vi "Read vision info keys.vi"() -> ()   [LabVIEW 2020]
panel:
  out "SpatialCalibrationY":T1
  out "error out":errorcluster
  out "Exposure":T1
  out "ROI":T2={"Width"={"Value"=618.0, "Min"=1.0, "Max"=3000.0, "StepSize"=1.0, "Tolerance"=0.0, "valueactual"=0.0}, "Height"={"Value"=813.0, "Min"=1.0, "Max"=3000.0, "StepSize"=1.0, "Tolerance"=0.0, "valueactual"=0.0}, "OffsetX"={"Value"=0.0, "Min"=0.0, "Max"=1000.0, "StepSize"=1.0, "Tolerance"=0.0, "valueactual"=0.0}, "OffsetY"={"Value"=0.0, "Min"=0.0, "Max"=1000.0, "StepSize"=1.0, "Tolerance"=0.0, "valueactual"=0.0}}
  out "SpatialCalibration":T1
  out "Keys":string[](array[string])
  in  "Image path":path
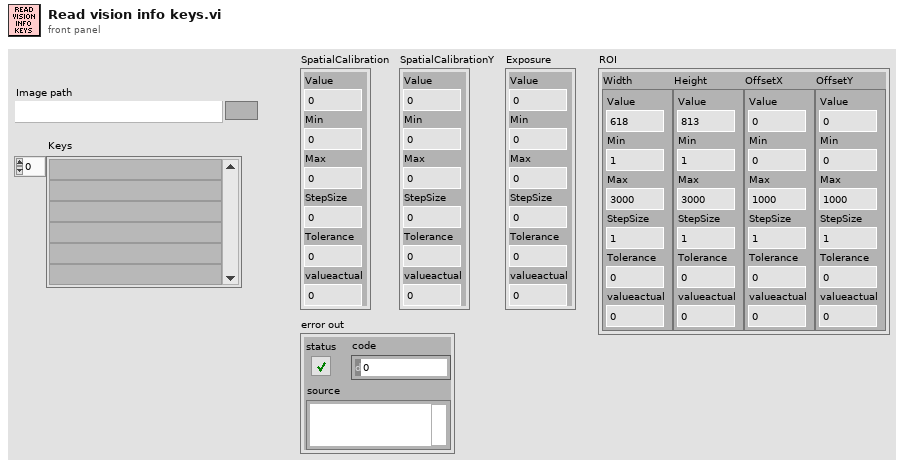
[diagram p1: front panel]
types:
  T1 = cluster{"Value":dbl, "Min":dbl, "Max":dbl, "StepSize":dbl, "Tolerance":dbl, "valueactual":dbl}
  T2 = cluster{"Width":cluster{"Value":dbl, "Min":dbl, "Max":dbl, "StepSize":dbl, "Tolerance":dbl, "valueactual":dbl}, "Height":cluster{"Value":dbl, "Min":dbl, "Max":dbl, "StepSize":dbl, "Tolerance":dbl, "valueactual":dbl}, "OffsetX":cluster{"Value":dbl, "Min":dbl, "Max":dbl, "StepSize":dbl, "Tolerance":dbl, "valueactual":dbl}, "OffsetY":cluster{"Value":dbl, "Min":dbl, "Max":dbl, "StepSize":dbl, "Tolerance":dbl, "valueactual":dbl}}
  T3 = cluster{"SpatialCalibration":cluster{"Value":dbl, "Min":dbl, "Max":dbl, "StepSize":dbl, "Tolerance":dbl, "valueactual":dbl}, "SpatialCalibrationY":cluster{"Value":dbl, "Min":dbl, "Max":dbl, "StepSize":dbl, "Tolerance":dbl, "valueactual":dbl}, "ROI":cluster{"Width":cluster{"Value":dbl, "Min":dbl, "Max":dbl, "StepSize":dbl, "Tolerance":dbl, "valueactual":dbl}, "Height":cluster{"Value":dbl, "Min":dbl, "Max":dbl, "StepSize":dbl, "Tolerance":dbl, "valueactual":dbl}, "OffsetX":cluster{"Value":dbl, "Min":dbl, "Max":dbl, "StepSize":dbl, "Tolerance":dbl, "valueactual":dbl}, "OffsetY":cluster{"Value":dbl, "Min":dbl, "Max":dbl, "StepSize":dbl, "Tolerance":dbl, "valueactual":dbl}}, "Exposure":cluster{"Value":dbl, "Min":dbl, "Max":dbl, "StepSize":dbl, "Tolerance":dbl, "valueactual":dbl}}
  T4 = typedef "IMAQ Image.ctl" = refnum<image>
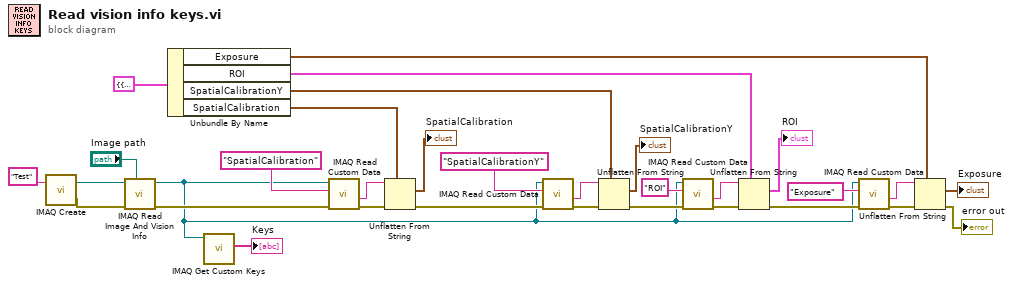
[diagram p0: block diagram]
diagram:
  n1 = call "IMAQ Create"("Image Name"="Test") -> ("New Image"=w30:T4, "error out"=w31:errorcluster)  [unwired: 4 in]
  n2 = call "IMAQ Read Image And Vision Info"("File Path"="Image path", "error in (no error)"=w31, "Image"=w30) -> ("error out"=w23:errorcluster, "Image Out"=w1:T4)  [unwired: 6 in, 1 out]
  n3 = Unbundle By Name(T3 {"SpatialCalibration"={"Value"=0.0, "Min"=0.0, "Max"=0.0, "StepSize"=0.0, "Tolerance"=0.0, "valueactual"=0.0}, "SpatialCalibrationY"={"Value"=0.0, "Min"=0.0, "Max"=0.0, "StepSize"=0.0, "Tolerance"=0.0, "valueactual"=0.0}, "ROI"={"Width"={"Value"=618.0, "Min"=1.0, "Max"=3000.0, "StepSize"=1.0, "Tolerance"=0.0, "valueactual"=0.0}, "Height"={"Value"=813.0, "Min"=1.0, "Max"=3000.0, "StepSize"=1.0, "Tolerance"=0.0, "valueactual"=0.0}, "OffsetX"={"Value"=0.0, "Min"=0.0, "Max"=1000.0, "StepSize"=1.0, "Tolerance"=0.0, "valueactual"=0.0}, "OffsetY"={"Value"=0.0, "Min"=0.0, "Max"=1000.0, "StepSize"=1.0, "Tolerance"=0.0, "valueactual"=0.0}}, "Exposure"={"Value"=0.0, "Min"=0.0, "Max"=0.0, "StepSize"=0.0, "Tolerance"=0.0, "valueactual"=0.0}}) -> ("Exposure"=w12:T1, "ROI"=w17:T2, "SpatialCalibrationY"=w4:T1, "SpatialCalibration"=w5:T1)
  n4 = call "IMAQ Get Custom Keys"("Image"=w1) -> ("Keys"=→"Keys":string[])  [unwired: 7 in, 3 out]
  n5 = call "IMAQ Read Custom Data"("error in (no error)"=w23, "Key"="SpatialCalibration", "Image"=w1) -> ("error out"=w27:errorcluster, "Custom Data Out"=w28:string)  [unwired: 6 in, 1 out]
  n6 = Unflatten From String(type=w5, binary string=w28, error in (no error)=w27) -> (value=→"SpatialCalibration":T1, error out=w6:errorcluster)  [unwired: 2 in, 1 out]
  n7 = call "IMAQ Read Custom Data"("error in (no error)"=w6, "Key"="SpatialCalibrationY", "Image"=w1) -> ("error out"=w9:errorcluster, "Custom Data Out"=w8:string)  [unwired: 6 in, 1 out]
  n8 = Unflatten From String(type=w4, binary string=w8, error in (no error)=w9) -> (value=→"SpatialCalibrationY":T1, error out=w2:errorcluster)  [unwired: 2 in, 1 out]
  n9 = call "IMAQ Read Custom Data"("error in (no error)"=w2, "Key"="ROI", "Image"=w1) -> ("error out"=w22:errorcluster, "Custom Data Out"=w21:string)  [unwired: 6 in, 1 out]
  n10 = Unflatten From String(type=w17, binary string=w21, error in (no error)=w22) -> (value=→"ROI":T2, error out=w13:errorcluster)  [unwired: 2 in, 1 out]
  n11 = call "IMAQ Read Custom Data"("error in (no error)"=w13, "Key"="Exposure", "Image"=w1) -> ("error out"=w14:errorcluster, "Custom Data Out"=w15:string)  [unwired: 6 in, 1 out]
  n12 = Unflatten From String(type=w12, binary string=w15, error in (no error)=w14) -> (value=→"Exposure":T1, error out=→"error out":errorcluster)  [unwired: 2 in, 1 out]
